vi "SetEC.vi"(1 "ecin100ns":u64=1, 2 "board_sel":u32=1) -> ()   [LabVIEW 2015]
uses:
  ESLSCDLL.dll
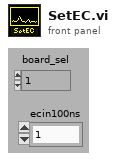
[diagram p1: front panel]
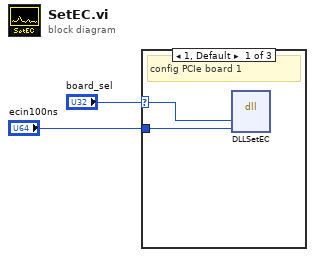
[diagram p0: block diagram]
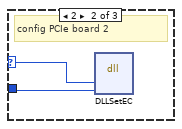
[diagram p2: hidden frame]
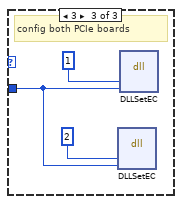
[diagram p3: hidden frame]
diagram:
  n1 = case shown="1, Default" "board_sel" {
    selector: "board_sel" -> [w3 w5 _]
    tunnel: "ecin100ns" -> [w4 w6 w7]
    frame 1, Default {
      # "config PCIe board 1"
      n2 = dll-call lib="C:/ENTW/PCIE/lv64/board.vis/ESLSCDLL.dll" fn="DLLSetEC" ("lwlscdll.dll:DLLSetTemp")("drv"=w3, "ecin100ns"=w4) -> ()  [unwired: 6 in, 2 out]
    }
    frame 2 {
      # "config PCIe board 2"
      n3 = dll-call lib="C:/ENTW/PCIE/lv64/board.vis/ESLSCDLL.dll" fn="DLLSetEC" ("lwlscdll.dll:DLLSetTemp")("drv"=w5, "ecin100ns"=w6) -> ()  [unwired: 6 in, 2 out]
    }
    frame 3 {
      # "config both PCIe boards"
      n4 = dll-call lib="C:/ENTW/PCIE/lv64/board.vis/ESLSCDLL.dll" fn="DLLSetEC" ("lwlscdll.dll:DLLSetTemp")("drv"=u32 2, "ecin100ns"=w7) -> ()  [unwired: 6 in, 2 out]
      n5 = dll-call lib="C:/ENTW/PCIE/lv64/board.vis/ESLSCDLL.dll" fn="DLLSetEC" ("lwlscdll.dll:DLLSetTemp")("drv"=u32 1, "ecin100ns"=w7) -> ()  [unwired: 6 in, 2 out]
    }
  }
